vi "ComputePodCostFunctions.vi"(4 "Default timestep":dbl, 5 "Desired Terminal State":T2, 6 "Pod State Data":T4, 7 "Cost Function Weights":T3, 8 "Pod Configuration":T5, 9 "Mass Subset":dbl, 10 "Potential Drive Magnitude Changes":dbl[](array[numeric]), 11 "Potential Turret Angle Changes":dbl[](array[numeric])) -> (1 "Drive Motor Data":T1, 2 "Turret Motor Data":T1, 3 "Optimal Solution":T3)   [LabVIEW 2014]
uses:
  Variables/Physical data.vi
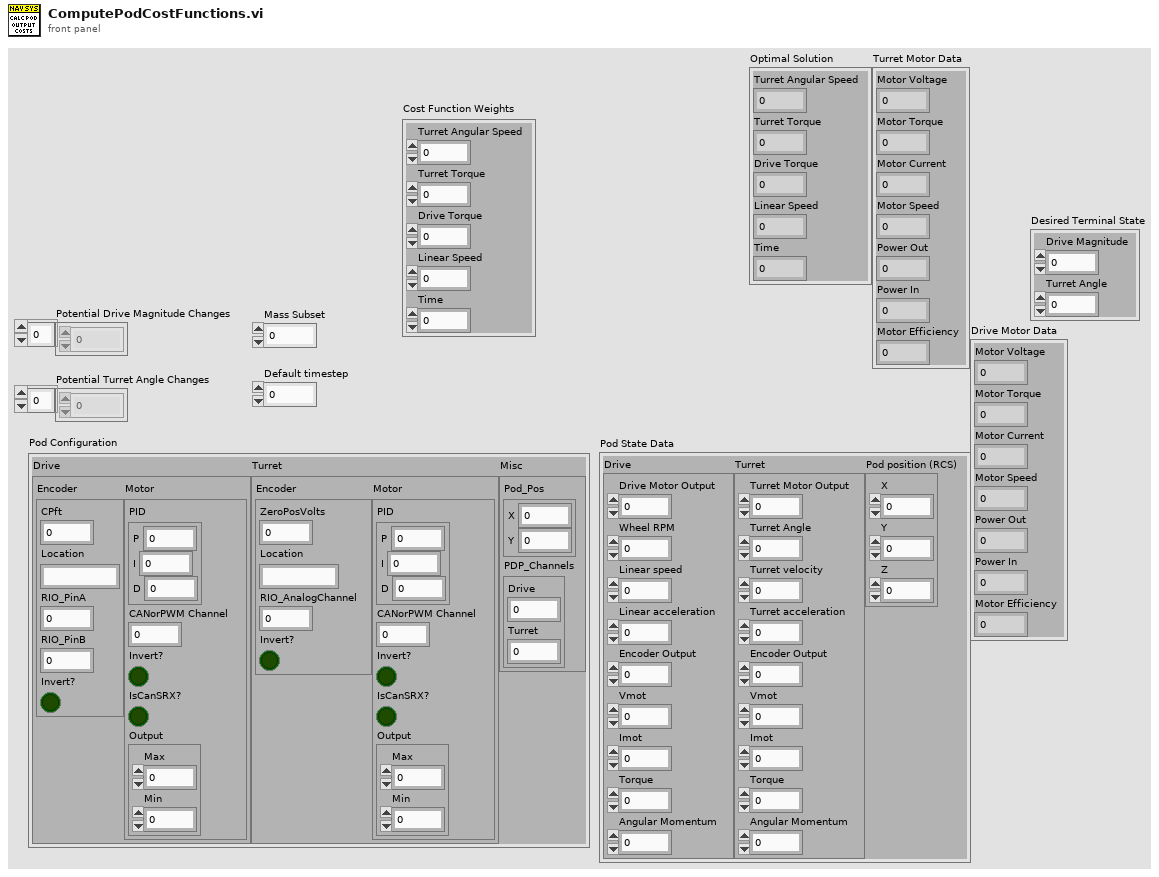
[diagram p1: front panel]
types:
  T1 = cluster{"Motor Voltage":dbl, "Motor Torque":dbl, "Motor Current":dbl, "Motor Speed":dbl, "Power Out":dbl, "Power In":dbl, "Motor Efficiency":dbl}
  T2 = cluster{"Drive Magnitude":dbl, "Turret Angle":dbl}
  T3 = cluster{"Turret Angular Speed":dbl, "Turret Torque":dbl, "Drive Torque":dbl, "Linear Speed":dbl, "Time":dbl}
  T4 = cluster{"Drive":cluster{"Drive Motor Output":dbl, "Wheel RPM":dbl, "Linear speed":dbl, "Linear acceleration":dbl, "Encoder Output":dbl, "Vmot":dbl, "Imot":dbl, "Torque":dbl, "Angular Momentum":dbl}, "Turret":cluster{"Turret Motor Output":dbl, "Turret Angle":dbl, "Turret velocity":dbl, "Turret acceleration":dbl, "Encoder Output":dbl, "Vmot":dbl, "Imot":dbl, "Torque":dbl, "Angular Momentum":dbl}, "Pod position (RCS)":cluster{"X":dbl, "Y":dbl, "Z":dbl}}
  T5 = cluster{"Drive":cluster{"Encoder":cluster{"CPft":dbl, "Location":string, "RIO_PinA":i32, "RIO_PinB":i32, "Invert?":bool}, "Motor":cluster{"PID":cluster{"P":dbl, "I":dbl, "D":dbl}, "CANorPWM Channel":i32, "Invert?":bool, "IsCanSRX?":bool, "Output":cluster{"Max":dbl, "Min":dbl}}}, "Turret":cluster{"Encoder":cluster{"ZeroPosVolts":dbl, "Location":string, "RIO_AnalogChannel":i32, "Invert?":bool}, "Motor":cluster{"PID":cluster{"P":dbl, "I":dbl, "D":dbl}, "CANorPWM Channel":i32, "Invert?":bool, "IsCanSRX?":bool, "Output":cluster{"Max":dbl, "Min":dbl}}}, "Misc":cluster{"Pod_Pos":cluster{"X":dbl, "Y":dbl}, "PDP_Channels":cluster{"Drive":i32, "Turret":i32}}}
  T6 = cluster{"Free Current":dbl, "Stall Current":dbl, "Stall Torque":dbl, "Free Speed":dbl, "Gear Ratio":dbl, "Efficiency":dbl, "Moment":dbl}
  T7 = cluster{"Motor Torque":dbl, "Motor Torque":dbl, "Motor Speed":dbl}
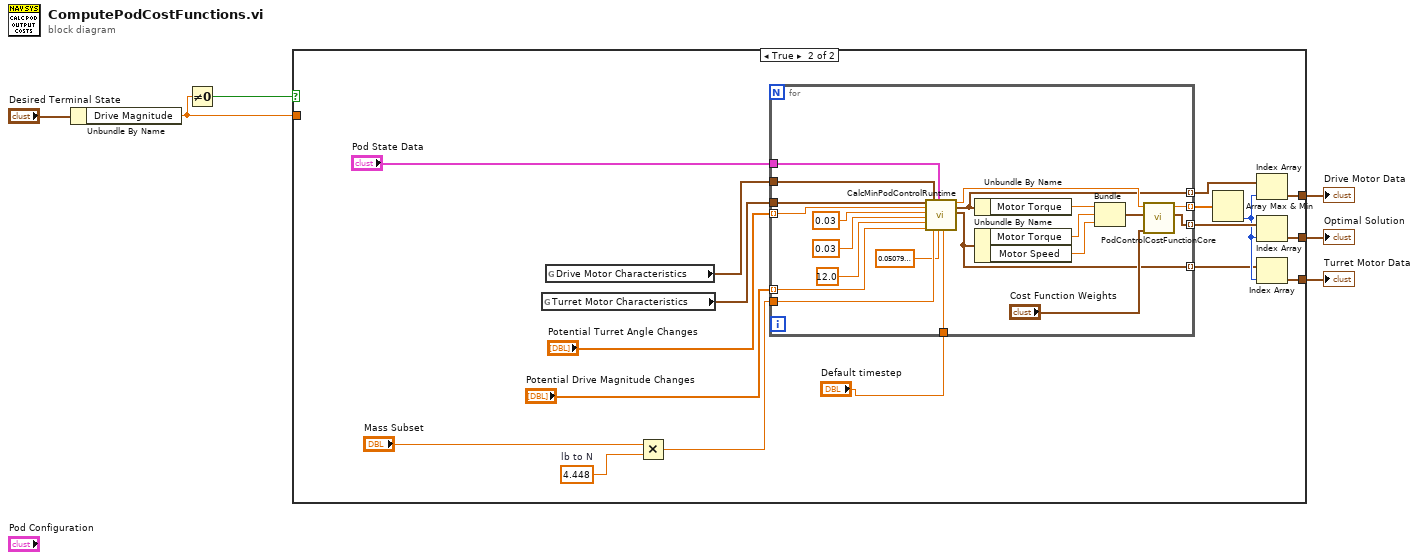
[diagram p0: block diagram]
diagram:
  n1 = Unbundle By Name("Desired Terminal State") -> ("Drive Magnitude"=w4:dbl)
  n2 = Not Equal To 0?(x=w4) -> (x != 0?=w1:bool)
  n3 = case shown="True" w1 {
    tunnel: [_ w14] -> w6
    tunnel: w4 -> [_ _]
    tunnel: [_ w10] -> w3
    tunnel: [_ w9] -> w2
    frame False {
      # "We don't want any outputs when the setpoint magnitude is zero,\nso disable the whole control algorithm"
    }
    frame True {
      w21 = 4.448  # lb to N
      n4 = global read "Physical data.vi" "Turret Motor Characteristics"() -> (w17:T6)
      n5 = global read "Physical data.vi" "Drive Motor Characteristics"() -> (w19:T6)
      n6 = Multiply(x="Mass Subset", y=w21) -> (x*y=w20:dbl)
      n7 = for {
        tunnel: "Potential Turret Angle Changes" -> [w36] mode=indexing
        tunnel: w20 -> [w40]
        tunnel: "Potential Drive Magnitude Changes" -> [w41] mode=indexing
        tunnel: w19 -> [w32]
        tunnel: w17 -> [w35]
        tunnel: [w43] -> w16 mode=indexing
        tunnel: [w42] -> w15 mode=indexing
        tunnel: [w27] -> w12 mode=indexing
        tunnel: [w26] -> w11 mode=indexing
        tunnel: "Pod State Data" -> [w25]
        tunnel: "Default timestep" -> [w24]
        n8 = call "CalcMinPodControlRuntime.vi"("Turret Motor Characteristics"=w35, "Turret Angle Change"=w36, "Wheel width (m)"=0.03, "Wheel Off-center dist (m)"=0.03, "Max Turret Motor Volts"=12.0, "Drive Magnitude Change"=w41, "Drive Motor Characteristics"=w32, "Mass Subset (N)"=w40, "Pod State Data"=w25, "Wheel radius"=0.050799999999999956, "Runtime"=w24) -> ("Min. Runtime"=w33:dbl, "Drive Motor Data"=w27:T1, "Turret Motor Data"=w26:T1)  [unwired: 6 in]
        n9 = Unbundle By Name(w27) -> ("Motor Torque"=w29:dbl)
        n10 = Unbundle By Name(w26) -> ("Motor Torque"=w30:dbl, "Motor Speed"=w31:dbl)
        n11 = Bundle("Motor Torque"=w29, "Motor Torque"=w30, "Motor Speed"=w31) -> (w28:T7)  [unwired: 1 in]
        n12 = call "PodControlCostFunctionCore.vi"("Cost Function Weights"="Cost Function Weights", "Output States"=w28, "Coerrected Timestep"=w33) -> ("All States Out"=w42:T3, "Cost"=w43:dbl)  [unwired: 7 in]
      }
      n13 = Array Max & Min(array=w16) -> (min index (indices)=w13:i32)  [unwired: 3 out]
      n14 = Index Array(array=w12, index=w13) -> (element=w9:T1)
      n15 = Index Array(array=w15, index=w13) -> (element=w14:T3)
      n16 = Index Array(array=w11, index=w13) -> (element=w10:T1)
    }
  }
  "Optimal Solution" <- w6
  "Turret Motor Data" <- w3
  "Drive Motor Data" <- w2
